vi "Meas Write Record Header File.vi"(4 "record segments info":T1[](array[typedef]), 6 "samples count":i64, 7 "corrections":T2 {"transducers"."channels"."Phase index" min=1 step=1}, 8 "error in":errorcluster, 9 "adc session":T5={"niScope"={"channel cfg"=[], "sessions"=[], "multi cards"=FALSE, "channels"=0, "type"=enum."n/a", "memory [B/chn]"=0, "ext. clock [Hz]"=0.0, "samples count"=0, "use streaming"=FALSE, "proc setup"={"packet size [smpl]"=0, "current timeout [s]"=0.0, "blk2blk timeout [s]"=0.0, "event time"=timestamp(0 s since 1904-01-01), "temp sampl T [s]"=0.0, "data queue"=refnum, "stop notifier"=refnum, "proc ref"=refnum}, "sample width [B]"=0, "ranges [V]"=[], "trigger setup"={"coupling"=1, "level [V]"=0.0, "slope"=0, "mode"=enum."Immediate"}, "fs [Hz]"=0.0, "bitres [bit]"=0, "clock source"=enum."VAL_NO_SOURCE"}, "3458A"={"channels"=[], "sync unit"={"VISA"="", "type"=enum."Picotest U6200A"}, "awg unit"={"type"=enum."Agilent 331xxA to 332xxA", "VISA"="", "enable 10MHz ref"=FALSE}, "sync mode"=enum."MASTER-SLAVE, MASTER clocked by TIMER", "streaming mode"=FALSE, "idn mode"=enum."Auto", "sampling mode"=enum."DCV", "Ts [s]"=0.0, "sample memory [B]"=0, "proc setup"={"channel id"=0, "packet size [smpl]"=0, "current timeout [s]"=0.0, "blk2blk timeout [s]"=0.0, "event time"=timestamp(0 s since 1904-01-01), "stop notifier"=refnum, "data queues"=[], "proc refs"=[], "bus semaphore"=refnum}, "sample size [B]"=0, "sample count"=0, "aux data"={"channel id"=0, "valid?"=[], "gain [V]"=[], "timestamp [s]"=[], "Ts [s]"=0.0, "abs timestamp"=timestamp(0 s since 1904-01-01), "t [deg C]"=[], "multiplex timestamp [s]"=-1.0, "only multiplex?"=FALSE, "multiplex smpl offset"=0}, "ranges [V]"=[], "aperture [s]"=0.0, "LEVEL trigger"={"edge"=enum."POS", "level [V]"=0.0, "coupling"=enum."DC"}, "trigger mode"=enum."AUTO", "measure temp.?"=FALSE, "disp mesages"=[], "shared bus?"=FALSE, "disable display?"=FALSE, "aper mode"=enum."Manual", "aper rules"=[], "multiplex"={"cycles"=0, "delay [s]"=0.0, "enabled"=FALSE, "overhead [s]"=1.0, "tot smpls"=0}}, "dsdll"={"dsdll"={"dsdll path"=path "", "dsdll handle"=[], "output devices"=[], "capture devices"=[]}, "channels"=0, "device id"=0, "channel idns"=[], "proc setup"={"packet size [smpl]"=0, "current timeout [s]"=0.0, "blk2blk timeout [s]"=0.0, "event time"=timestamp(0 s since 1904-01-01), "data queue"=refnum, "stop notifier"=refnum, "proc ref"=refnum}, "samples count"=0, "fs [Hz]"=0.0}, "type"=enum."niScope", "channel idn str"=[], "aux instr idn str"=[], "modified?"=FALSE, "simadc"={"channels"=[], "range [V]"=0.0, "Ts step [s]"=0.0, "time [s]"=0.0, "fs [Hz]"=0.0, "count"=0, "smpl offset"=0, "set count"=0, "bit res"=0}, "force rst?"=FALSE, "exit mode"=enum."Immediate reset", "exit dly"=0.0, "exit tmr"=timestamp(0 s since 1904-01-01), "busy?"=FALSE, "accessed?"=FALSE, "multiplex"={"Type"=enum."Dummy", "gen com ssn"={"visa"="", "primary"=enum."None", "secondary"=enum."None", "channels"=[]}, "delay before [s]"=0.0, "delay post [s]"=0.0, "sequence"=[], "enabled"=FALSE, "ref timestamp [s]"=0.0, "idn string"="", "dev niScope"="", "niScope idx"=0}} {"3458A"."channels"."Range [Vpk]" min=0.0; "niScope"."trigger setup"."level [V]" format="%.2f"; "niScope"."trigger setup"."coupling" items=["AC"=0, "DC"=1, "HF Reject"=3, "LF Reject"=4, "AC Plus HF Reject"=1001]; "niScope"."channel cfg"."Range [Vpk]" min=0.0; "niScope"."channel cfg"."Channel" min=0}, 10 "aux data":T54, 11 "sequence item":T50) -> (0 "error out":errorcluster)   [LabVIEW 2013]
doc: "Write logged temperature data to the samples MAT file. It will write the data even if they are empty."
uses:
  adc/ADC Aux Data.ctl
  Meas Sequence Item.ctl
  Meas Sampling Configuration.ctl
  adc/ADC Trig Config.ctl
  adc/ADC Trig Mode Source.ctl
  adc/ADC Trig Coupling.ctl
  adc/ADC Trig Slope.ctl
  processing/QWTB/Meas Proc QWTB Algorithm Parameter Data.ctl
  adc/ADC Session.ctl
  drivers/niScope/niScope Session.ctl
  drivers/niScope/niScope Virtual Channel Config.ctl
  drivers/niScope/niScope Virtual Channel Mode.ctl
  drivers/niScope/niScope Virtual Channel Input Z.ctl
  drivers/niScope/niScope Virtual Channel Coupling.ctl
  drivers/niScope/niScope Type.ctl
  drivers/niScope/niScope Digitizing Process Options.ctl
  drivers/niScope/niScope Data Packet.ctl
  drivers/niScope/niScope Trigger Setup.ctl
  <instrlib>/niScope/Controls/niScope trigger coupling.ctl
  <instrlib>/niScope/Controls/niScope trigger slope.ctl
  drivers/niScope/niScope Reference Clock.ctl
  drivers/DMM/3458A Digitizer Session.ctl
  drivers/DMM/3458A Virtual Channel Config.ctl
  drivers/Counter/Counter Session.ctl
  drivers/Counter/Counter Type.ctl
  drivers/AWG/AWG Session.ctl
  drivers/AWG/AWG Type.ctl
  drivers/DMM/3458A Sync Mode.ctl
  drivers/DMM/3458A Idn Mode.ctl
  drivers/DMM/3458A Digitizing Low Levels/Configure/Sampling Mode.ctl
  drivers/DMM/3458A Digitizing Process Options.ctl
  drivers/DMM/3458A Data Packet.ctl
  drivers/DMM/3458A Aux Record Data.ctl
  drivers/DMM/3458A Digitizing Low Levels/Configure/Level Setup.ctl
  drivers/DMM/3458A Digitizing Low Levels/Configure/First Sample Trigger.ctl
  drivers/DMM/3458A Aperture Selection Mode.ctl
  drivers/DMM/3458A Multiplexing Config.ctl
  drivers/dsdll/DSDLL Session.ctl
  drivers/dsdll/dsdll.lvlibp/dsdll_instance.ctl
  drivers/dsdll/dsdll.lvlibp/dsdll_device_record.ctl
  drivers/dsdll/DSDLL Process Config.ctl
  drivers/dsdll/DSDLL Data Packet.ctl
  adc/ADC Type.ctl
  drivers/simulated_adc/SimAdc Config.ctl
  drivers/simulated_adc/SimAdc Channel Cfg.ctl
  adc/ADC On Close Action.ctl
  adc/Multiplexer/MPX Session.ctl
  adc/Multiplexer/MPX Type.ctl
  drivers/Multiplexers/Generic COM/GCOMM Session.ctl
  drivers/Multiplexers/Generic COM/GCOMM Signal.ctl
  drivers/Multiplexers/Generic COM/GCOMM Virtual Channel.ctl
  drivers/Multiplexers/Generic COM/GCOMM Logic State.ctl
  Corrections/Corr Setup.ctl
  Corrections/Corr Tranducer Item.ctl
  Corrections/Corr Digitizers.ctl
  adc/Multiplexer/MPX Record Segment Info.ctl
  <vilib>/Analysis/baseanly.llb/Mean (DBL).vi
  octave/infolib.lvlibp/Private/Add matrix polymorph parts/1D String.vi
  octave/infolib.lvlibp/Private/Add key polymorph parts/I64.vi
  octave/infolib.lvlibp/Private/Add key polymorph parts/String.vi
  octave/infolib.lvlibp/Private/Add key polymorph parts/Boolean.vi
  octave/infolib.lvlibp/Private/Get key polymorph parts/GetI64.vi
  octave/infolib.lvlibp/Private/Add key polymorph parts/EXT.vi
  octave/infolib.lvlibp/Private/Add matrix polymorph parts/2D EXT.vi
  octave/infolib.lvlibp/Private/Add matrix polymorph parts/2D String.vi
  octave/infolib.lvlibp
  <vilib>/Analysis/NI_AALBase.lvlib
  drivers/niScope/niScope Virtual Digitizer.lvlib
  drivers/DMM/3458A Virtual Digitizer.lvlib
  drivers/Counter/Counter.lvlib
  drivers/AWG/AWG.lvlib
  drivers/DMM/3458A Digitizing Low Levels/3458A Digitizing Low Levels.lvlib
  drivers/dsdll/dsdll.lvlibp
  drivers/dsdll/DSDLL Virtual Digitizer.lvlib
panel:
  in  "coupling":T47
  in  "slope":T48
  in  "source":T49
  # "ADC:"
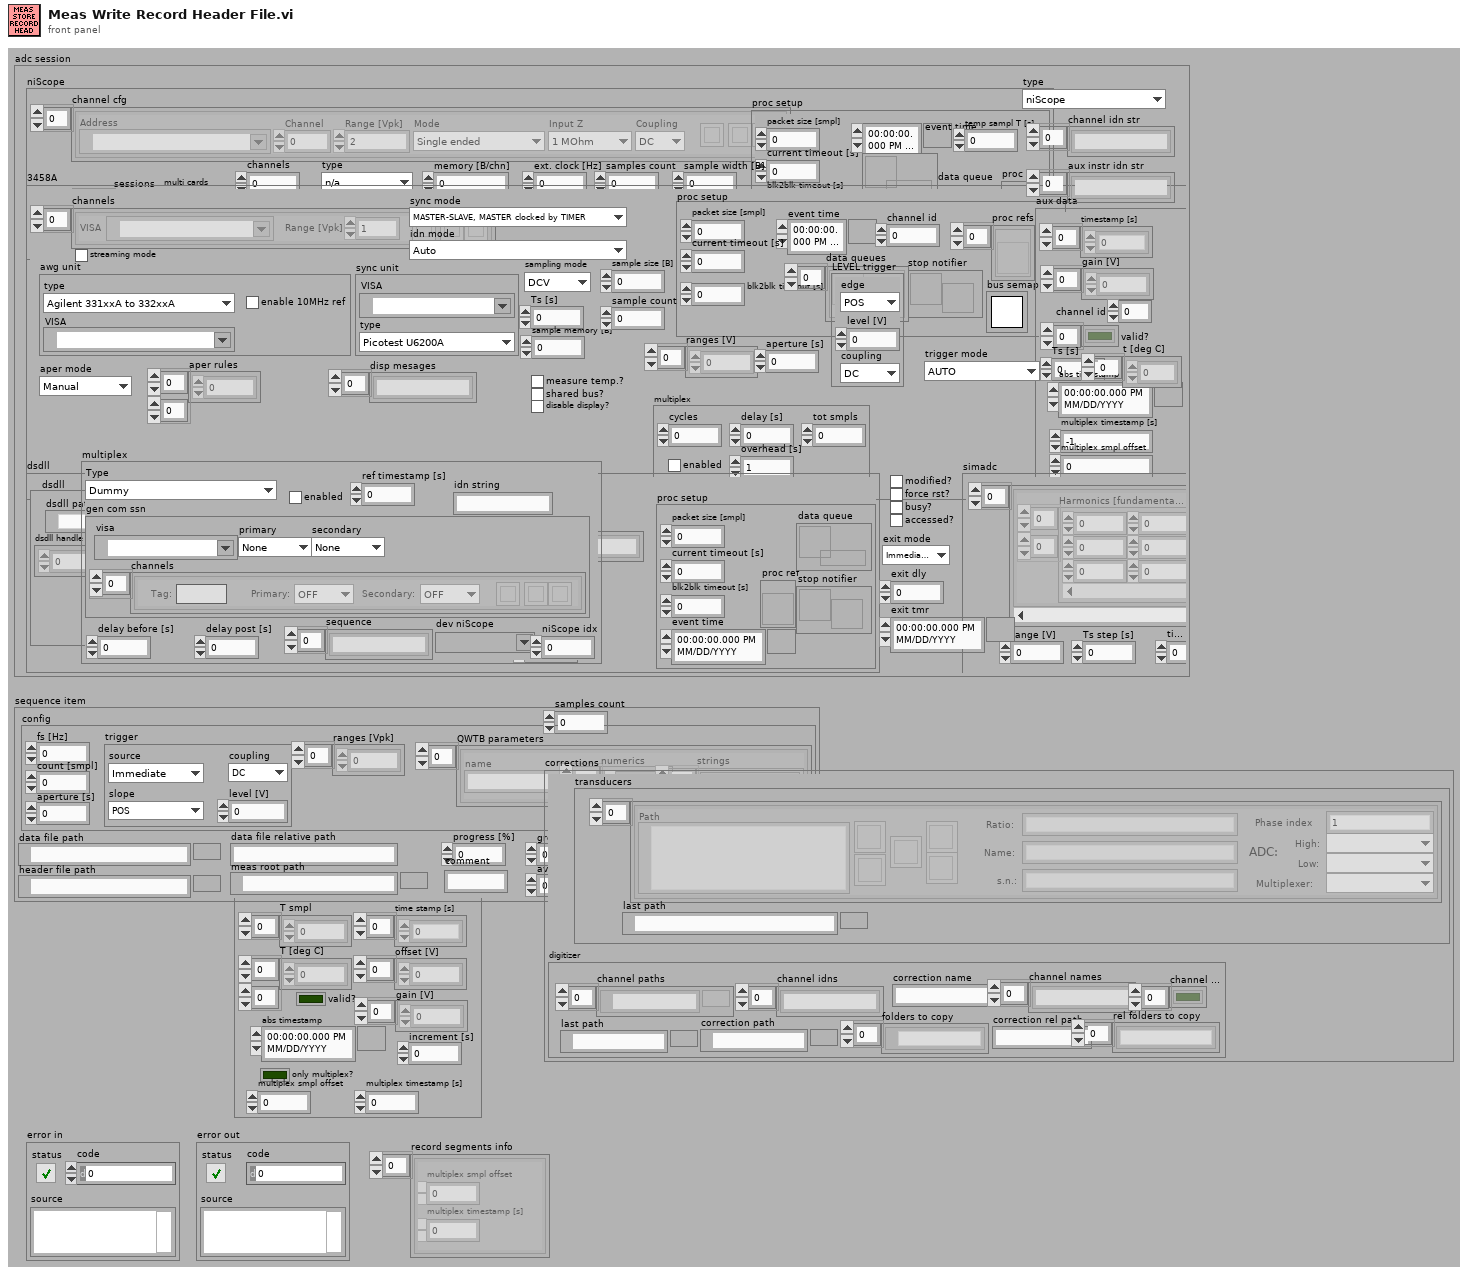
[diagram p1: front panel]
types:
  T1 = typedef "MPX Record Segment Info.ctl" = cluster{"multiplex smpl offset":i64, "multiplex timestamp [s]":dbl}
  T2 = typedef "Corr Setup.ctl" = cluster{"transducers":cluster{"channels":T3[], "last path":path}, "digitizer":T4}
  T3 = typedef "Corr Tranducer Item.ctl" = cluster{"Path":path, "Ratio:":string, "Name:":string, "btn rem":bool, "btn up":bool, "btn down":bool, "s.n.:":string, "btn open":bool, "ratio o/i":dbl, "chn hi":u16, "chn lo":u16, "Phase index":i32, "btn edit":bool, "mpx chn":u16}
  T4 = typedef "Corr Digitizers.ctl" = cluster{"last path":path, "channel paths":path[], "channel idns":string[], "correction name":string, "channel names":string[], "folders to copy":path[], "channel valid":bool[], "correction path":path, "correction rel path":string, "rel folders to copy":string[]}
  T5 = typedef "ADC Session.ctl" = cluster{"niScope":T6, "3458A":T17, "dsdll":T33, "type":T37, "channel idn str":string[], "aux instr idn str":string[], "modified?":bool, "simadc":T38, "force rst?":bool, "exit mode":T40, "exit dly":dbl, "exit tmr":timestamp, "busy?":bool, "accessed?":bool, "multiplex":T41}
  T6 = typedef "niScope Virtual Digitizer.lvlib/niScope Session.ctl" = cluster{"channel cfg":T7[], "sessions":refnum<k20>[], "multi cards":bool, "channels":i32, "type":T11, "memory [B/chn]":i32, "ext. clock [Hz]":dbl, "samples count":i64, "use streaming":bool, "proc setup":T12, "sample width [B]":i32, "ranges [V]":dbl[], "trigger setup":T13, "fs [Hz]":dbl, "bitres [bit]":i32, "clock source":T16}
  T7 = typedef "niScope Virtual Digitizer.lvlib/niScope Virtual Channel Config.ctl" = cluster{"Address":refnum<k15>, "Channel":i32, "Mode":T8, "Input Z":T9, "Coupling":T10, "Range [Vpk]":dbl, "btn clr":bool, "btn up":bool, "btn down":bool}
  T8 = typedef "niScope Virtual Digitizer.lvlib/niScope Virtual Channel Mode.ctl" = enum16{"Single ended", "Unbal. differential", "Differential"}
  T9 = typedef "niScope Virtual Digitizer.lvlib/niScope Virtual Channel Input Z.ctl" = enum16{"1 MOhm", "50 Ohm"}
  T10 = typedef "niScope Virtual Digitizer.lvlib/niScope Virtual Channel Coupling.ctl" = enum16{"AC", "DC", "GND"}
  T11 = typedef "niScope Virtual Digitizer.lvlib/niScope Type.ctl" = enum16{"n/a", "5922"}
  T12 = typedef "niScope Virtual Digitizer.lvlib/niScope Digitizing Process Options.ctl" = cluster{"packet size [smpl]":i64, "current timeout [s]":dbl, "blk2blk timeout [s]":dbl, "event time":timestamp, "temp sampl T [s]":dbl, "data queue":refnum<queue>, "stop notifier":refnum<notifier>, "proc ref":refnum<vi>}
  T13 = typedef "niScope Virtual Digitizer.lvlib/niScope Trigger Setup.ctl" = cluster{"coupling":T14, "level [V]":dbl, "slope":T15, "mode":enum16{"Immediate", "External", "Level"}}
  T14 = typedef "niScope trigger coupling.ctl" = u16
  T15 = typedef "niScope trigger slope.ctl" = i32
  T16 = typedef "niScope Virtual Digitizer.lvlib/niScope Reference Clock.ctl" = enum16{"VAL_NO_SOURCE", "VAL_CLK_IN", "VAL_PXI_CLOCK", "VAL_EXTERNAL"}
  T17 = typedef "3458A Virtual Digitizer.lvlib/3458A Digitizer Session.ctl" = cluster{"channels":T18[], "sync unit":T19, "awg unit":T21, "sync mode":T23, "streaming mode":bool, "idn mode":T24, "sampling mode":T25, "Ts [s]":dbl, "sample memory [B]":i32, "proc setup":T26, "sample size [B]":i32, "sample count":i32, "aux data":T28, "ranges [V]":dbl[], "aperture [s]":dbl, "LEVEL trigger":T29, "trigger mode":T30, "measure temp.?":bool, "disp mesages":string[], "shared bus?":bool, "disable display?":bool, "aper mode":T31, "aper rules":dbl[][], "multiplex":T32}
  T18 = typedef "3458A Virtual Digitizer.lvlib/3458A Virtual Channel Config.ctl" = cluster{"VISA":refnum<visa-resource-name>, "Range [Vpk]":dbl, "btn clr":bool, "btn up":bool, "btn down":bool}
  T19 = typedef "Counter.lvlib/Counter Session.ctl" = cluster{"VISA":refnum<visa-resource-name>, "type":T20}
  T20 = typedef "Counter.lvlib/Counter Type.ctl" = enum16{"Picotest U6200A", "dummy"}
  T21 = typedef "AWG.lvlib/AWG Session.ctl" = cluster{"type":T22, "VISA":refnum<visa-resource-name>, "enable 10MHz ref":bool}
  T22 = typedef "AWG.lvlib/AWG Type.ctl" = enum16{"Agilent 331xxA to 332xxA", "Agilent 335xxA to 336xxA", "Tektronix AFG3101C", "dummy"}
  T23 = typedef "3458A Virtual Digitizer.lvlib/3458A Sync Mode.ctl" = enum16{"MASTER-SLAVE, MASTER clocked by TIMER", "MASTER-SLAVE, MASTER clocked by AWG", "ALL clocked by AWG", "MASTER-SLAVE, ALL clocked by TIMER", "ALL clocked by AWG with DFLL"}
  T24 = typedef "3458A Virtual Digitizer.lvlib/3458A Idn Mode.ctl" = enum16{"Auto", "Sequential (chn A, chn B, ...)", "From calibration string"}
  T25 = typedef "3458A Virtual Digitizer.lvlib/3458A Digitizing Low Levels.lvlib/Sampling Mode.ctl" = enum16{"DCV", "DSDC", "DSAC"}
  T26 = typedef "3458A Virtual Digitizer.lvlib/3458A Digitizing Process Options.ctl" = cluster{"channel id":i32, "packet size [smpl]":i32, "current timeout [s]":dbl, "blk2blk timeout [s]":dbl, "event time":timestamp, "stop notifier":refnum<notifier>, "data queues":refnum<queue>[], "proc refs":refnum<vi>[], "bus semaphore":T27}
  T27 = typedef "Semaphore RefNum" = refnum<k1>
  T28 = typedef "3458A Virtual Digitizer.lvlib/3458A Aux Record Data.ctl" = cluster{"channel id":i32, "valid?":bool[], "gain [V]":dbl[], "timestamp [s]":dbl[], "Ts [s]":dbl, "abs timestamp":timestamp, "t [deg C]":dbl[], "multiplex timestamp [s]":dbl, "only multiplex?":bool, "multiplex smpl offset":i64}
  T29 = typedef "3458A Virtual Digitizer.lvlib/3458A Digitizing Low Levels.lvlib/Level Setup.ctl" = cluster{"edge":enum16{"POS", "NEG"}, "level [V]":dbl, "coupling":enum16{"DC", "AC"}}
  T30 = typedef "3458A Virtual Digitizer.lvlib/3458A Digitizing Low Levels.lvlib/First Sample Trigger.ctl" = enum16{"AUTO", "EXT", "SYN", "SGL", "HOLD", "LEVEL"}
  T31 = typedef "3458A Virtual Digitizer.lvlib/3458A Aperture Selection Mode.ctl" = enum16{"Manual", "Maximum", "Table"}
  T32 = typedef "3458A Multiplexing Config.ctl" = cluster{"cycles":i32, "delay [s]":dbl, "enabled":bool, "overhead [s]":dbl, "tot smpls":i64}
  T33 = typedef "DSDLL Virtual Digitizer.lvlib/DSDLL Session.ctl" = cluster{"dsdll":T34, "channels":i32, "device id":i32, "channel idns":string[], "proc setup":T36, "samples count":i32, "fs [Hz]":dbl}
  T34 = typedef "dsdll.lvlibp/dsdll_instance.ctl" = cluster{"dsdll path":path, "dsdll handle":u8[], "output devices":T35[], "capture devices":T35[]}
  T35 = typedef "dsdll.lvlibp/dsdll_device_record.ctl" = cluster{"guid":u8[], "name":string}
  T36 = typedef "DSDLL Virtual Digitizer.lvlib/DSDLL Process Config.ctl" = cluster{"packet size [smpl]":i32, "current timeout [s]":dbl, "blk2blk timeout [s]":dbl, "event time":timestamp, "data queue":refnum<queue>, "stop notifier":refnum<notifier>, "proc ref":refnum<vi>}
  T37 = typedef "ADC Type.ctl" = enum16{"niScope", "3458A", "DirectSound DLL", "dummy"}
  T38 = typedef "SimAdc Config.ctl" = cluster{"channels":T39[], "range [V]":dbl, "Ts step [s]":dbl, "time [s]":dbl, "fs [Hz]":dbl, "count":i64, "smpl offset":i64, "set count":i64, "bit res":i32}
  T39 = typedef "SimAdc Channel Cfg.ctl" = cluster{"harmonics":dbl[][], "btn clear":bool, "noise":dbl, "fundamental [Hz]":dbl}
  T40 = typedef "ADC On Close Action.ctl" = enum16{"Immediate reset", "Delayed reset"}
  T41 = typedef "MPX Session.ctl" = cluster{"Type":T42, "gen com ssn":T43, "delay before [s]":dbl, "delay post [s]":dbl, "sequence":string[], "enabled":bool, "ref timestamp [s]":dbl, "idn string":string, "dev niScope":refnum<k15>, "niScope idx":i32}
  T42 = typedef "MPX Type.ctl" = enum16{"Dummy", "Generic - COM port", "Generic - niScope PFI"}
  T43 = typedef "GCOMM Session.ctl" = cluster{"visa":refnum<visa-resource-name>, "primary":T44, "secondary":T44, "channels":T45[]}
  T44 = typedef "GCOMM Signal.ctl" = enum16{"None", "DTR", "RTS"}
  T45 = typedef "GCOMM Virtual Channel.ctl" = cluster{"Primary:":T46, "Secondary:":T46, "btn clr":bool, "btn up":bool, "btn down":bool, "Tag:":string}
  T46 = typedef "GCOMM Logic State.ctl" = enum16{"OFF", "ON"}
  T47 = typedef "ADC Trig Coupling.ctl" = enum16{"DC", "AC"}
  T48 = typedef "ADC Trig Slope.ctl" = enum16{"POS", "NEG"}
  T49 = typedef "ADC Trig Mode Source.ctl" = enum16{"Immediate", "External", "Level"}
  T50 = typedef "Meas Sequence Item.ctl" = cluster{"config":T51, "data file path":path, "header file path":path, "group id":i32, "average id":i32, "group done?":bool, "adc modified?":bool, "source modified?":bool, "progress [%]":dbl, "groups cnt":i32, "average cnt":i32, "data file relative path":string, "meas root path":path, "calculate?":bool, "comment":string}
  T51 = typedef "Meas Sampling Configuration.ctl" = cluster{"fs [Hz]":dbl, "count [smpl]":i64, "aperture [s]":dbl, "trigger":T52, "ranges [Vpk]":dbl[], "QWTB parameters":T53[]}
  T52 = typedef "ADC Trig Config.ctl" = cluster{"source":T49, "level [V]":dbl, "coupling":T47, "slope":T48}
  T53 = typedef "Meas Proc QWTB Algorithm Parameter Data.ctl" = cluster{"name":string, "numerics":dbl[], "strings":string[]}
  T54 = typedef "ADC Aux Data.ctl" = cluster{"offset [V]":dbl[], "gain [V]":dbl[], "time stamp [s]":dbl[], "increment [s]":dbl, "T smpl":i64[], "T [deg C]":dbl[][], "valid?":bool, "abs timestamp":timestamp, "only multiplex?":bool, "multiplex smpl offset":i64, "multiplex timestamp [s]":dbl}
  T55 = typedef "ADC Capabilities.ctl" = cluster{"max samples count":i64, "max fs [Hz]":ext, "min fs [Hz]":ext, "Ts step [s]":ext, "max Ts [s]":ext, "min Ts [s]":ext, "allows streaming?":bool, "streaming on?":bool, "has level trig?":bool, "has ext trig?":bool, "has aperture?":bool, "aper min [s]":dbl, "aper max [s]":dbl, "channels count":i32, "has ranges?":bool, "has temperature?":bool, "has temperature log?":bool, "has selfcal?":bool, "fs step [Hz]":ext, "smpl rate step mode":T56}
  T56 = typedef "ADC Sampling Rate Step Mode.ctl" = enum16{"const period", "const frequency"}
  T57 = typedef "ADC Attribute.ctl" = cluster{"name":string, "value":string[], "is constant per group":bool}
  T58 = typedef "ADC Current Configuration.ctl" = cluster{"count [smpl]":i64, "channels count":i32, "fs [Hz]":dbl, "ranges [V]":dbl[], "trigger":T52, "ext freq. locked?":bool, "streaming on?":bool, "is int16?":bool, "bitres":i32}
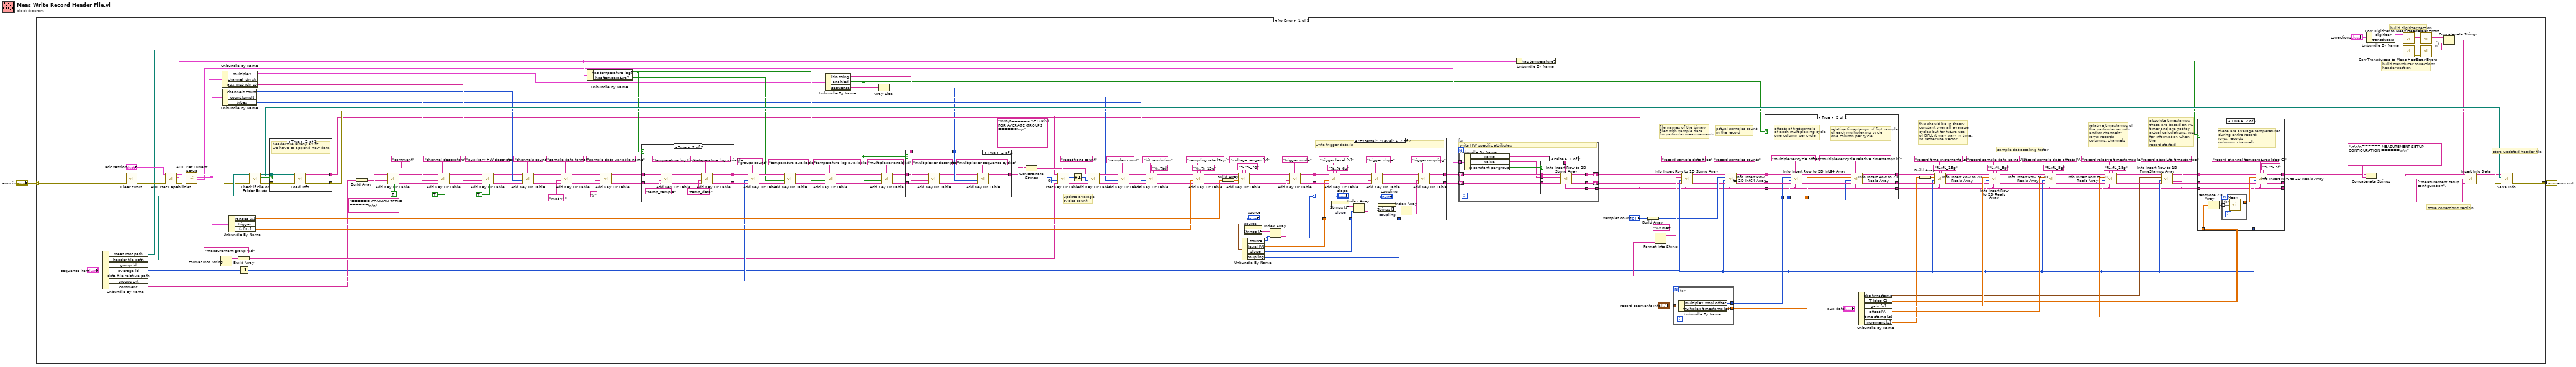
[diagram p0: block diagram]
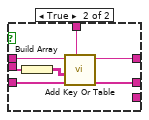
[diagram p6: hidden frame]
diagram:
  n1 = case shown="No Error" "error in" {
    selector: "error in" -> [w124 w287]
    tunnel: [w156 w287] -> w2
    frame No Error {
      w154 = "repetitions count" ("key description")
      # "store corrections section"
      # "build digitizer section"
      # "build transducer corrections\nheader section"
      # "actual samples count\nin the record"
      # "absolute timestamps\nthese are based on PC\ntimer and are not for \nactual calculations, just\nfor information when the\nrecord started"
      # "file names of the binary\nfiles with sample data\nfor particular measurements"
      # "relative timestamps of\nthe particular records\nand/or channels:\nrows: records\ncolumns: channels"
      # "sample dat ascaling factor"
      # "this should be in theory\nconstant over all average\ncycles but for future use\nof DFLL it may vary in time,\nso rather use vector"
      # "update average\ncycles count"
      # "store updated header file"
      n2 = Unbundle By Name("sequence item") -> ("meas root path"=w56:path, "header file path"=w63:path, "group id"=w75:i32, "average id"=w149:i32, "data file relative path"=w62:string, "groups cnt"=w74:i32, "comment"=w28:string)
      n3 = call <vilib>:"Clear Errors.vi"("error in (no error)"=w124) -> ("error out"=w102:errorcluster)  [unwired: 6 in]
      n4 = call "ADC Get Capabilities.vi"("error in"=w102, "adc session in"="adc session") -> ("error out"=w103:errorcluster, "capabilities"=w79:T55, "adc session out"=w100:T5)  [unwired: 7 in]
      n5 = call "ADC Get Current Setup.vi"("error in"=w103, "adc session in"=w100) -> ("error out"=w51:errorcluster, "device specific attributes"=w17:T57[], "common attributes"=w109:T58, "adc session out"=w132:T5)  [unwired: 6 in]
      n6 = Format Into String(format string="measurement group %d", w75) -> (resulting string=w134:string)  [unwired: 2 in, 1 out]
      n7 = Unbundle By Name(w132) -> ("multiplex"=w16:T41, "channel idn str"=w44:string[], "aux instr idn str"=w128:string[])
      n8 = Unbundle By Name(w109) -> ("channels count"=w115:i32, "count [smpl]"=w86:i64, "bitres"=w35:i32)
      n9 = Unbundle By Name(w109) -> ("ranges [V]"=w108:dbl[], "trigger"=w107:T52, "fs [Hz]"=w106:dbl)
      n10 = Build Array(w134) -> (w52:string[])
      n11 = Decrement(x=w149) -> (x-1=w20:i32)
      n12 = call <vilib>:"Check if File or Folder Exists.vi"("error in (no error)"=w51, "path"=w63) -> ("error out"=w179:errorcluster, "file or folder exists?"=w180:bool, "dup path"=w158:path)  [unwired: 7 in]
      n13 = case shown="True" w180 {
        tunnel: w179 -> [w282 w286]
        tunnel: w158 -> [_ w285]
        tunnel: [_ w284] -> w18
        tunnel: [w282 w283] -> w157
        frame False {
          # "no header file exit\nstart new one"
        }
        frame True {
          # "header file alrady exist\nwe have to append new data"
          n14 = call "Load Info.vi"("error in"=w286, "filename"=w285) -> ("error out"=w283:errorcluster, "info data"=w284:string)  [unwired: 8 in]
        }
      }
      n15 = Build Array(w28) -> (w27:string[])
      n16 = call-poly "Add Key Or Table.vi"("column vector (F)"=TRUE, "key description"="comment", "string"=w27, "info data"="====== COMMON SETUP ======\n\n" ("string")) -> ("sections out"=w32:string[], "info data out"=w31:string)  [unwired: 6 in]
      n17 = call-poly "Add Key Or Table.vi"("column vector (F)"=TRUE, "key description"="channel descriptors", "sections"=w32, "string"=w44, "info data"=w31) -> ("sections out"=w131:string[], "info data out"=w130:string)  [unwired: 5 in]
      n18 = call-poly "Add Key Or Table.vi"("column vector (F)"=TRUE, "key description"="auxiliary HW descriptors", "sections"=w131, "string"=w128, "info data"=w130) -> ("sections out"=w14:string[], "info data out"=w13:string)  [unwired: 5 in]
      n19 = call-poly "Add Key Or Table.vi"("key description"="channels count", "sections"=w14, "numeric"=w115, "info data"=w13) -> ("sections out"=w122:string[], "info data out"=w121:string)  [unwired: 6 in]
      n20 = call-poly "Add Key Or Table.vi"("key description"="sample data format", "sections"=w122, "string"="mat-v4" ("multi-line string"), "info data"=w121) -> ("sections out"=w85:string[], "info data out"=w84:string)  [unwired: 6 in]
      n21 = Unbundle By Name(w79) -> ("has temperature log?"=w65:bool, "has temperature?"=w64:bool)
      n22 = call-poly "Add Key Or Table.vi"("key description"="sample data variable name", "sections"=w85, "string"="y", "info data"=w84) -> ("sections out"=w81:string[], "info data out"=w80:string)  [unwired: 6 in]
      n23 = case shown="True" w65 {
        tunnel: w81 -> [w210 w219]
        tunnel: w80 -> [w211 w218]
        tunnel: [w211 w214] -> w77
        tunnel: [w210 w212] -> w78
        frame False {
        }
        frame True {
          n24 = call-poly "Add Key Or Table.vi"("key description"="temperature log time stamp variable name", "sections"=w219, "string"="temp_sample", "info data"=w218) -> ("sections out"=w216:string[], "info data out"=w213:string)  [unwired: 6 in]
          n25 = call-poly "Add Key Or Table.vi"("key description"="temperature log variable name", "sections"=w216, "string"="temp_data", "info data"=w213) -> ("sections out"=w212:string[], "info data out"=w214:string)  [unwired: 6 in]
        }
      }
      n26 = call-poly "Add Key Or Table.vi"("key description"="groups count", "sections"=w78, "numeric"=w74, "info data"=w77) -> ("sections out"=w68:string[], "info data out"=w66:string)  [unwired: 6 in]
      n27 = call-poly "Add Key Or Table.vi"("key description"="temperature available", "sections"=w68, "boolean"=w64, "info data"=w66) -> ("sections out"=w67:string[], "info data out"=w69:string)  [unwired: 6 in]
      n28 = call-poly "Add Key Or Table.vi"("key description"="temperature log available", "sections"=w67, "boolean"=w65, "info data"=w69) -> ("sections out"=w6:string[], "info data out"=w7:string)  [unwired: 6 in]
      n29 = Unbundle By Name(w16) -> ("idn string"=w15:string, "enabled"=w4:bool, "sequence"=w11:string[])
      n30 = Array Size(array=w11) -> (size(s)=w10:i32)
      n31 = call-poly "Add Key Or Table.vi"("key description"="multiplexer enabled", "sections"=w6, "boolean"=w4, "info data"=w7) -> ("sections out"=w8:string[], "info data out"=w9:string)  [unwired: 6 in]
      n32 = case shown="True" w4 {
        tunnel: w15 -> [_ w205]
        tunnel: w10 -> [_ w203]
        tunnel: w9 -> [w197 w202]
        tunnel: w8 -> [_ w201]
        tunnel: [w197 w198] -> w5
        frame False {
        }
        frame True {
          n33 = call-poly "Add Key Or Table.vi"("key description"="multiplexer descriptor", "sections"=w201, "string"=w205, "info data"=w202) -> ("sections out"=w200:string[], "info data out"=w199:string)  [unwired: 6 in]
          n34 = call-poly "Add Key Or Table.vi"("key description"="multiplexer sequence cycles", "sections"=w200, "numeric"=w203, "info data"=w199) -> ("info data out"=w198:string)  [unwired: 6 in, 1 out]
        }
      }
      n35 = Concatenate Strings(w5, "\n\n\n====== SETUP(S) FOR AVERAGE GROUPS ======\n\n" ("string")) -> (w127:string)
      n36 = call-poly "Get Key Or Table.vi"("key description"=w154, "sections"=w52, "numeric"=i64 0, "info data"=w18) -> ("sections out"=w155:string[], "value"=w153:i64)  [unwired: 4 in, 2 out]
      n37 = Increment(x=w153) -> (x+1=w152:i64)
      n38 = call-poly "Add Key Or Table.vi"("key description"=w154, "sections"=w155, "numeric"=w152, "info data"=w127) -> ("sections out"=w89:string[], "info data out"=w88:string)  [unwired: 6 in]
      n39 = call-poly "Add Key Or Table.vi"("key description"="samples count", "sections"=w89, "numeric"=w86, "info data"=w88) -> ("sections out"=w39:string[], "info data out"=w36:string)  [unwired: 6 in]
      n40 = call-poly "Add Key Or Table.vi"("format string (%_20d)"="%.;%d" ("format string (%_20f)"), "key description"="bit resolution", "sections"=w39, "numeric"=w35, "info data"=w36) -> ("sections out"=w38:string[], "info data out"=w37:string)  [unwired: 5 in]
      n41 = call-poly "Add Key Or Table.vi"("format string (%_20f)"="%.;%_15g", "key description"="sampling rate [Sa/s]", "sections"=w38, "numeric"=w106, "info data"=w37) -> ("sections out"=w111:string[], "info data out"=w110:string)  [unwired: 5 in]
      n42 = Build Array(w108) -> (w116:dbl[][])
      n43 = call-poly "Add Key Or Table.vi"("format string (%_20f)"="%.;%_3g", "key description"="voltage ranges [V]", "sections"=w111, "numeric"=w116, "info data"=w110) -> ("sections out"=w119:string[], "info data out"=w120:string)  [unwired: 5 in]
      n44 = Unbundle By Name(w107) -> ("source"=w140:T49, "level [V]"=w138:dbl, "slope"=w137:T48, "coupling"=w136:T47)
      n45 = property on="source" class="Enum (strict)"() -> ("Strings []"=w142:string[])  [unwired: 2 in, 2 out]
      n46 = Index Array(array=w142, index=w140) -> (element=w141:string)
      n47 = call-poly "Add Key Or Table.vi"("key description"="trigger mode", "sections"=w119, "string"=w141, "info data"=w120) -> ("sections out"=w139:string[], "info data out"=w135:string)  [unwired: 6 in]
      n48 = case shown="\"External\", \"Level\"" w140 {
        tunnel: w139 -> [w262 w281]
        tunnel: w138 -> [_ w278]
        tunnel: w137 -> [_ w274]
        tunnel: w136 -> [_ w269]
        tunnel: [w262 w265] -> w105
        tunnel: [w261 w264] -> w104
        tunnel: w135 -> [w261 w263]
        frame Default {
        }
        frame "External", "Level" {
          # "write trigger details"
          n49 = call-poly "Add Key Or Table.vi"("format string (%_20f)"="%.;%_6g", "key description"="trigger level [V]", "sections"=w281, "numeric"=w278, "info data"=w263) -> ("sections out"=w276:string[], "info data out"=w267:string)  [unwired: 5 in]
          n50 = property on="slope" class="Enum (strict)"() -> ("Strings []"=w275:string[])  [unwired: 2 in, 2 out]
          n51 = Index Array(array=w275, index=w274) -> (element=w273:string)
          n52 = call-poly "Add Key Or Table.vi"("key description"="trigger slope", "sections"=w276, "string"=w273, "info data"=w267) -> ("sections out"=w271:string[], "info data out"=w266:string)  [unwired: 6 in]
          n53 = property on="coupling" class="Enum (strict)"() -> ("Strings []"=w270:string[])  [unwired: 2 in, 2 out]
          n54 = Index Array(array=w270, index=w269) -> (element=w268:string)
          n55 = call-poly "Add Key Or Table.vi"("key description"="trigger coupling", "sections"=w271, "string"=w268, "info data"=w266) -> ("sections out"=w265:string[], "info data out"=w264:string)  [unwired: 6 in]
        }
      }
      n56 = for {
        tunnel: w17 -> [w246] mode=indexing
        shift-right: [w245] -> w72
        shift-left: w105 -> [w242]
        shift-right: [w244] -> w50
        shift-left: w104 -> [w243]
        tunnel: w18 -> [w238]
        # "write HW specific attributes"
        n57 = Unbundle By Name(w246) -> ("name"=w241:string, "value"=w239:string[], "is constant per group"=w240:bool)
        n58 = case shown="False" w240 {
          tunnel: [w252 w260] -> w245
          tunnel: [w251 w259] -> w244
          tunnel: w243 -> [w250 w258]
          tunnel: w242 -> [w253 w257]
          tunnel: w241 -> [w249 w256]
          tunnel: w239 -> [w248 w254]
          tunnel: w238 -> [w247 _]
          frame False {
            n59 = call "Info Insert Row to 2D String Array.vi"("source info data"=w247, "key description"=w249, "sections in"=w253, "row to insert"=w248, "info data in"=w250) -> ("sections out"=w252:string[], "info data out"=w251:string)  [unwired: 5 in]
          }
          frame True {
            n60 = Build Array(w254) -> (w255:string[][])
            n61 = call-poly "Add Key Or Table.vi"("key description"=w256, "sections"=w257, "string"=w255, "info data"=w258) -> ("sections out"=w260:string[], "info data out"=w259:string)  [unwired: 6 in]
          }
        }
      }
      n62 = Unbundle By Name(w79) -> ("has temperature?"=w94:bool)
      n63 = Build Array("samples count") -> (w112:i64[])
      n64 = Format Into String(format string="%s.mat", w62) -> (resulting string=w146:string)  [unwired: 2 in, 1 out]
      n65 = for {
        tunnel: "record segments info" -> [w209] mode=indexing
        tunnel: [w208] -> w23 mode=indexing
        tunnel: [w207] -> w19 mode=indexing
        n66 = Unbundle By Name(w209) -> ("multiplex smpl offset"=w208:i64, "multiplex timestamp [s]"=w207:dbl)
      }
      n67 = call "Info Insert Row to 1D String Array.vi"("source info data"=w18, "key description"="record sample data files", "sections in"=w72, "row index to insert"=w20, "string to insert"=w146, "info data in"=w50) -> ("sections out"=w90:string[], "info data out"=w91:string)  [unwired: 4 in]
      n68 = call "Info Insert Row to 2D Int64 Array.vi"("source info data"=w18, "key description"="record samples counts", "sections in"=w90, "row index to insert"=w20, "row to insert"=w112, "info data in"=w91) -> ("sections out"=w26:string[], "info data out"=w25:string)  [unwired: 4 in]
      n69 = case shown="True" w4 {
        tunnel: w26 -> [w184 w196]
        tunnel: w25 -> [w183 w195]
        tunnel: w23 -> [_ w193]
        tunnel: [w183 w189] -> w22
        tunnel: [w184 w188] -> w21
        tunnel: w20 -> [_ w187]
        tunnel: w19 -> [_ w186]
        tunnel: w18 -> [w182 w185]
        tunnel: [w182 w185] -> w3
        frame False {
        }
        frame True {
          # "relative timestamps of first sample\nof each multiplexing cycle\none column per cycle"
          # "offsets of first sample\nof each multiplexing cycle\none column per cycle"
          n70 = call "Info Insert Row to 2D Int64 Array.vi"("source info data"=w185, "key description"="multiplexer cycle offsets", "sections in"=w196, "row index to insert"=w187, "row to insert"=w193, "info data in"=w195) -> ("sections out"=w191:string[], "info data out"=w190:string)  [unwired: 4 in]
          n71 = call "Info Insert Row to 2D Reals Array.vi"("source info data"=w185, "key description"="multiplexer cycle relative timestamps [s]", "sections in"=w191, "row index to insert"=w187, "row to insert"=w186, "info data in"=w190) -> ("sections out"=w188:string[], "info data out"=w189:string)  [unwired: 4 in]
        }
      }
      n72 = Unbundle By Name("aux data") -> ("abs timestamp"=w92:timestamp, "T [deg C]"=w93:dbl[][], "gain [V]"=w176:dbl[], "offset [V]"=w170:dbl[], "time stamp [s]"=w165:dbl[], "increment [s]"=w160:dbl)
      n73 = Build Array(w160) -> (w159:dbl[])
      n74 = call "Info Insert Row to 2D Reals Array.vi"("format string (%_20f)"="%.;%_15g", "source info data"=w3, "key description"="record time increments [s]", "sections in"=w21, "row index to insert"=w20, "row to insert"=w159, "info data in"=w22) -> ("sections out"=w162:string[], "info data out"=w161:string)  [unwired: 3 in]
      n75 = call "Info Insert Row to 2D Reals Array.vi"("format string (%_20f)"="%.;%_8g", "source info data"=w3, "key description"="record sample data gains [V]", "sections in"=w162, "row index to insert"=w20, "row to insert"=w176, "info data in"=w161) -> ("sections out"=w172:string[], "info data out"=w171:string)  [unwired: 3 in]
      n76 = call "Info Insert Row to 2D Reals Array.vi"("format string (%_20f)"="%.;%_8g", "source info data"=w3, "key description"="record sample data offsets [V]", "sections in"=w172, "row index to insert"=w20, "row to insert"=w170, "info data in"=w171) -> ("sections out"=w167:string[], "info data out"=w166:string)  [unwired: 3 in]
      n77 = call "Info Insert Row to 2D Reals Array.vi"("format string (%_20f)"="%.;%_18g", "source info data"=w3, "key description"="record relative timestamps [s]", "sections in"=w167, "row index to insert"=w20, "row to insert"=w165, "info data in"=w166) -> ("sections out"=w99:string[], "info data out"=w98:string)  [unwired: 3 in]
      n78 = call "Info Insert Row to 1D TimeStamps Array.vi"("source info data"=w3, "key description"="record absolute timestamps", "sections in"=w99, "row index to insert"=w20, "timestamp to insert"=w92, "info data in"=w98) -> ("sections out"=w96:string[], "info data out"=w95:string)  [unwired: 4 in]
      n79 = case shown="True" w94 {
        tunnel: w96 -> [w223 w235]
        tunnel: w20 -> [_ w233]
        tunnel: w3 -> [w222 w226]
        tunnel: w95 -> [w224 w232]
        tunnel: [w223 w231] -> _
        tunnel: [w224 w230] -> w34
        tunnel: [w222 w226] -> _
        tunnel: w93 -> [_ w228]
        frame False {
        }
        frame True {
          # "these are average temperatures\nduring entire record:\nrows: records\ncolumns: channels"
          n80 = Transpose 2D Array(2D array=w228) -> (transposed array=w225:dbl[][])
          n81 = for {
            tunnel: w225 -> [w237] mode=indexing
            tunnel: [w236] -> w227 mode=indexing
            n82 = call-poly <vilib>:"Mean.vi"("X"=w237) -> ("mean"=w236:dbl)  [unwired: 1 out]
          }
          n83 = call "Info Insert Row to 2D Reals Array.vi"("format string (%_20f)"="%.;%.3f", "source info data"=w226, "key description"="record channel temperatures [deg C]", "sections in"=w235, "row index to insert"=w233, "row to insert"=w227, "info data in"=w232) -> ("sections out"=w231:string[], "info data out"=w230:string)  [unwired: 3 in]
        }
      }
      n84 = Concatenate Strings(w34, "\n\n\n====== MEASUREMENT SETUP CONFIGURATION ======\n\n" ("string")) -> (w57:string)
      n85 = Unbundle By Name("corrections") -> ("digitizer"=w53:T4, "transducers"=w55:cluster{"channels":T3[], "last path":path})
      n86 = call "Corr Digitizer to Meas Header.vi"("digitizer in"=w53) -> ("error out"=w54:errorcluster, "info data out"=w48:string)  [unwired: 8 in, 1 out]
      n87 = call "Corr Transducers to Meas Header.vi"("measurement root path"=w56, "transducers in"=w55) -> ("error out"=w60:errorcluster, "info data out"=w46:string)  [unwired: 7 in, 1 out]
      n88 = call <vilib>:"Clear Errors.vi"("error in (no error)"=w54) -> ()  [unwired: 6 in, 1 out]
      n89 = call <vilib>:"Clear Errors.vi"("error in (no error)"=w60) -> ()  [unwired: 6 in, 1 out]
      n90 = Concatenate Strings(w48, "\n" ("string"), w46) -> (w47:string)
      n91 = call "Insert Info Data.vi"("info data to insert"=w47, "sections"=string[] ["measurement setup configuration"], "info data"=w57) -> ("info data out"=w49:string)  [unwired: 7 in, 1 out]
      n92 = call "Save Info.vi"("error in"=w157, "filename"=w158, "info data"=w49) -> ("error out"=w156:errorcluster)  [unwired: 8 in]
    }
    frame Error {
    }
  }
  "error out" <- w2
